vi "Set all voltage limits (SubVI).vi"() -> (3 "String":string)   [LabVIEW 2018]
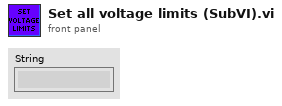
[diagram p1: front panel]
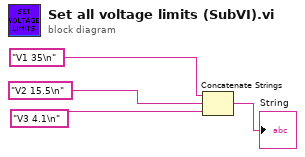
[diagram p0: block diagram]
diagram:
  n1 = Concatenate Strings("V1 35\n", "V2 15.5\n", "V3 4.1\n") -> (→"String":string)
